vi "Stop SmartMotor.vi"(0 "reference in":refnum<class "SmartMotor.lvclass">, 5 "error in (no error)":errorcluster) -> (14 "reference out":refnum<class "SmartMotor.lvclass">, 19 "error out":errorcluster)   [LabVIEW 2017, in "SmartMotor.lvclass"]
uses:
  SmartMotor.lvclass
  utils/SmartMotor Status.ctl
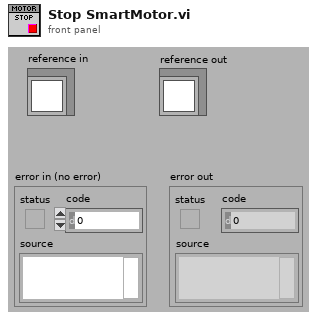
[diagram p1: front panel]
types:
  T1 = typedef "SmartMotor.lvclass/SmartMotor Status.ctl" = enum8{"Stopped", "Moving"}
  T2 = typedef "SmartMotor.lvclass/ObjectAttributes.ctl" = cluster{"SmartMotor Chain VISA Resource":refnum<visa-resource-name>, "SmartMotor Chain Address":i16, "Motor Absolute Position":i32, "Motor Relative Position":i32, "Motor Torque":i32, "Motor Voltage":i32, "Screwdriver Engaged":bool, "Screwdriver Torque Limit":i32, "Torque Monitor On/Off Status":bool, "Torque Monitor VI Reference":refnum<vi>, "Absolute Motor Torque (Filtered)":dbl, "SmartMotor Status":T1, "SmartMotor Error":T3}
  T3 = typedef "SmartMotor.lvclass/SmartMotor Error.ctl" = enum8{"None", "Read Error", "Low Voltage"}
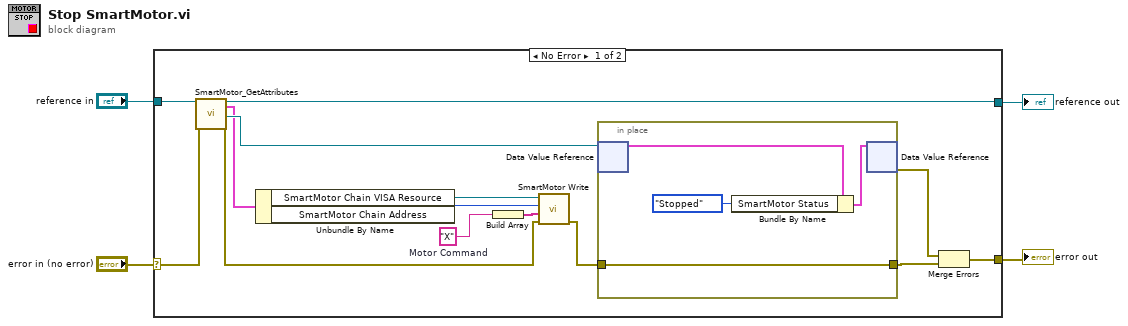
[diagram p0: block diagram]
diagram:
  n1 = case shown="No Error" "error in (no error)" {
    selector: "error in (no error)" -> [w17 w24]
    tunnel: [w15 w24] -> w3
    tunnel: [w16 w23] -> w1
    tunnel: "reference in" -> [w18 w23]
    frame No Error {
      w11 = "X"  # Motor Command
      n2 = call "SmartMotor_GetAttributes.vi"("reference in"=w18, "error in (no error)"=w17) -> ("reference out"=w16:refnum<class "SmartMotor.lvclass">, "Data"=w8:T2, "DataRef"=w14:refnum<data-value>, "error out"=w6:errorcluster)  [unwired: 14 in]
      n3 = Unbundle By Name(w8) -> ("SmartMotor Chain VISA Resource"=w10:refnum<visa-resource-name>, "SmartMotor Chain Address"=w9:i16)
      n4 = Build Array(w11) -> (w12:string[])
      n5 = call "SmartMotor Write.vi"("VISA resource IN"=w10, "Motor Number"=w9, "Motor Command Array"=w12, "Error In"=w6) -> ("Error Out"=w5:errorcluster)  [unwired: 3 in, 2 out]
      n6 = in-place {
        in-place-border: w5 -> [w19]
        in-place-border: [w19] -> w7
        n7 = in-place-dvr #1(w14) -> (w22:T2)  [unwired: 1 out]
        n8 = Bundle By Name(cluster=w22, "SmartMotor Status"=SmartMotor_Status."Stopped") -> (w21:T2)
        n9 = in-place-dvr #1(w21) -> (w13:errorcluster)  [unwired: 1 out]
      }
      n10 = Merge Errors(w13, w7) -> (w15:errorcluster)
    }
    frame Error {
    }
  }
  "error out" <- w3
  "reference out" <- w1
